vi "hari 2.vi"() -> ()   [LabVIEW 2020]
panel:
  out "Array":i32[](array[numeric])
  out "Numeric":i32
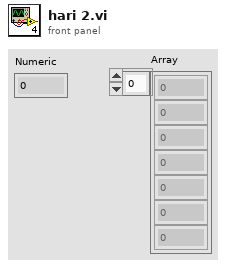
[diagram p1: front panel]
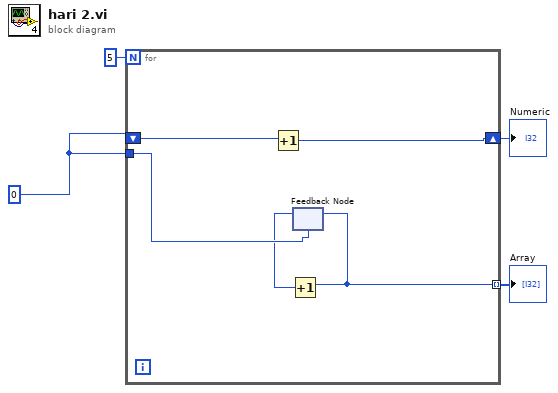
[diagram p0: block diagram]
diagram:
  w2 = 0
  n1 = for {
    N: 5 -> [_]
    shift-right: [w9] -> w3
    shift-left: w2 -> [w8]
    tunnel: w2 -> [w7]
    tunnel: [w5] -> w1 mode=indexing
    n2 = Increment(x=w8) -> (x+1=w9:i32)
    n3 = feedback #1(w7) -> (w6:i32)
    n4 = Increment(x=w6) -> (x+1=w5:i32)
    n5 = feedback-in #1(w5) -> ()
  }
  "Numeric" <- w3
  "Array" <- w1
